vi "AlternativeLauncher.vi"() -> ()   [LabVIEW 2013]
panel:
  out "2nd letter":string
  out "1st letter":string
  out "PASSWORD":string
  out "2nd":bool
  out "1st":bool
  out "Input Signal Energy":dbl
  out "Utterance":dbl[](graph)
  out "Slide":i32(slide) scale=0.0..3000.0
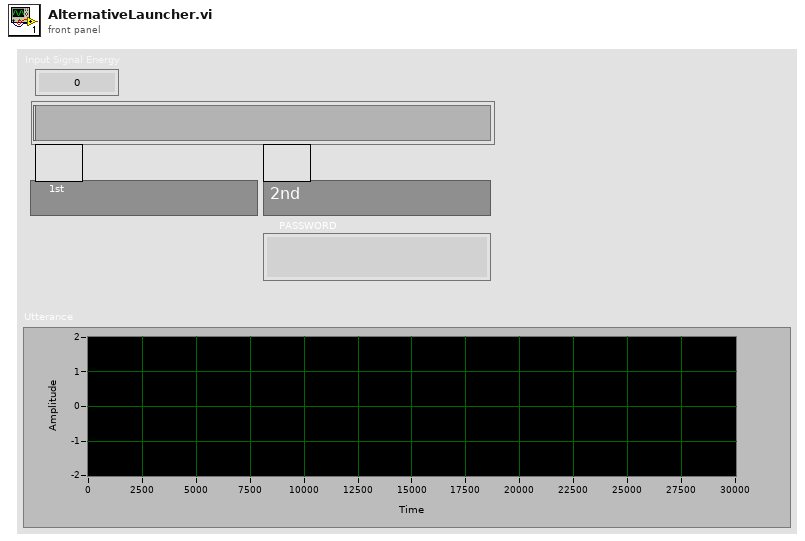
[diagram p1: front panel]
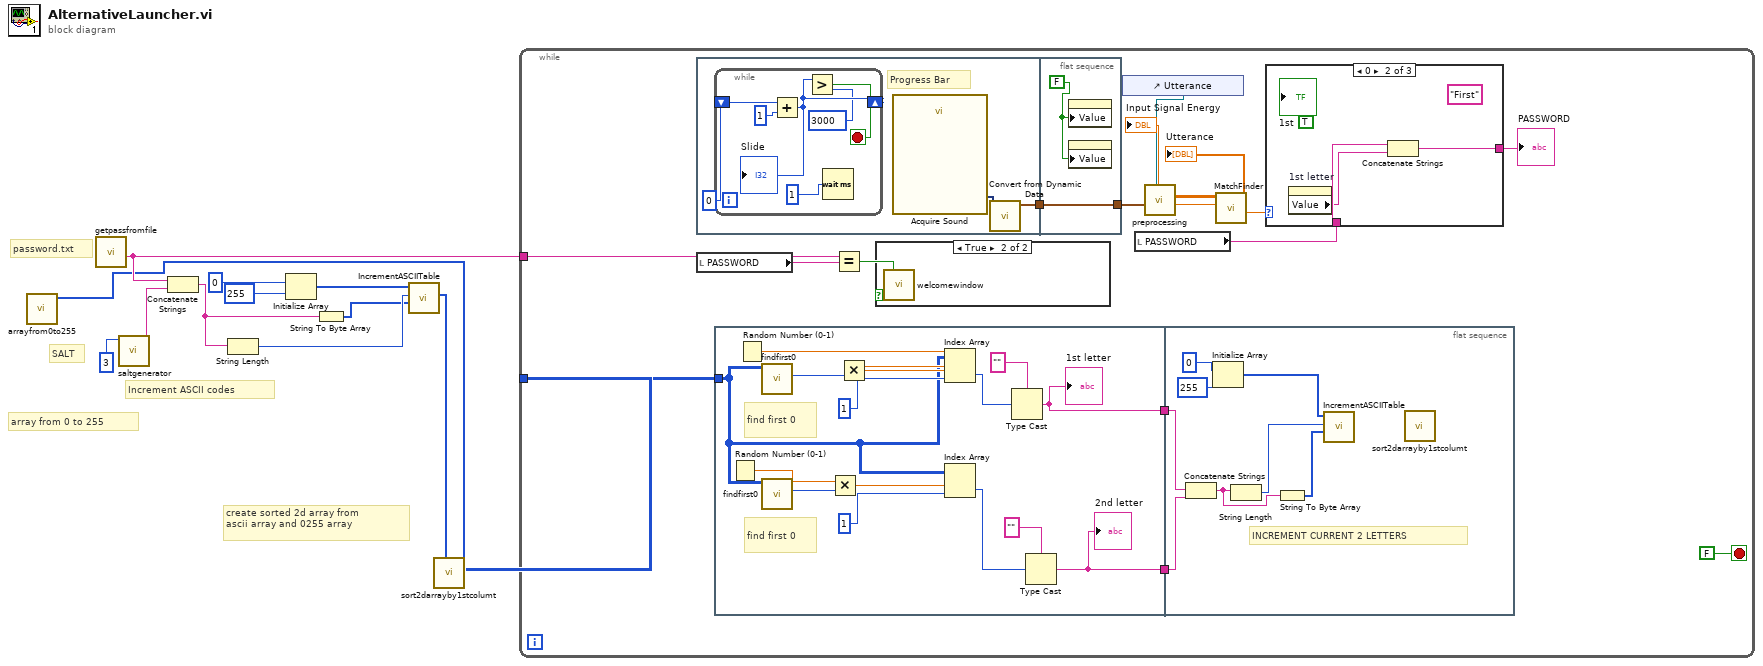
[diagram p0: block diagram]
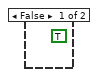
[diagram p2: hidden frame]
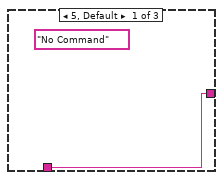
[diagram p3: hidden frame]
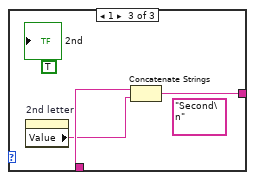
[diagram p4: hidden frame]
diagram:
  # "array from 0 to 255"
  # "create sorted 2d array from \nascii array and 0255 array"
  # "Increment ASCII codes"
  # "SALT"
  # "password.txt"
  n1 = call "arrayfrom0to255.vi"() -> ("Array 2"=w2:i32[])  [unwired: 11 in]
  n2 = call "getpassfromfile.vi"() -> ("line string"=w11:string)  [unwired: 11 in]
  n3 = call "saltgenerator.vi"("Numeric"=3) -> ("string"=w10:string)  [unwired: 10 in]
  n4 = Concatenate Strings(w11, w10) -> (w5:string)
  n5 = String Length(string=w5) -> (length=w6:i32)
  n6 = Initialize Array(0 ("dimension size"), 255 ("dimension size")) -> (w3:i32[])
  n7 = String To Byte Array(string=w5) -> (unsigned byte array=w4:u8[])
  n8 = call "IncrementASCIITable.vi"("0255array"=w4, "Numeric"=w6, "Array in"=w3) -> ("we array"=w9:i32[])  [unwired: 7 in, 1 out]
  n9 = call "sort2darrayby1stcolumt.vi"("array"=w2, "we array"=w9) -> ("Array"=w1:i32[][])  [unwired: 9 in]
  n10 = while {
    tunnel: w11 -> [w18]
    tunnel: w1 -> [w15]
    stop <- FALSE stop-if-true
    n11 = flat-sequence {
      tunnel: [w62] -> w23
      tunnel: [w72] -> w24
      tunnel: w23 -> [w72]
      frame #0 {
        # "Progress Bar"
        n12 = while {
          shift-right: [w67] -> _
          shift-left: 0 -> [w70]
          stop <- w65 stop-if-true
          n13 = Add(x=w70, y=1) -> (x+y=w67:i32)
          "Slide" <- w67
          n14 = Greater?(x=w67, y=u32 3000) -> (0:w65:bool)
          n15 = Wait (ms)(milliseconds to wait=u32 1) -> ()  [unwired: 1 out]
        }
        n16 = call "Acquire Sound"() -> ("Data"=w63:dynamicdata)  [unwired: 18 in, 1 out]
        n17 = call "Convert from Dynamic Data"("Dynamic Data Type"=w63) -> ("Array of Waveform"=w62:waveform(dbl)[])  [unwired: 3 in]
      }
      frame #1 {
        w71 = FALSE ("1st")
        n18 = property class="Bool (strict)"("Value"=w71) -> ()  [unwired: 2 in, 2 out]
        n19 = property class="Bool (strict)"("Value"=w71) -> ()  [unwired: 2 in, 2 out]
      }
    }
    n20 = local read "PASSWORD"() -> (w19:string)
    n21 = flat-sequence {
      tunnel: w15 -> [w36]
      tunnel: [w31] -> w14
      tunnel: [w30] -> w13
      tunnel: w14 -> [w47]
      tunnel: w13 -> [w46]
      frame #0 {
        # "find first 0"
        # "find first 0"
        n22 = Random Number (0-1)() -> (number: 0 to 1=w37:dbl)
        n23 = Random Number (0-1)() -> (number: 0 to 1=w44:dbl)
        n24 = call "findfirst0.vi"("Array"=w36) -> ("index of element"=w43:i32)  [unwired: 10 in]
        n25 = call "findfirst0.vi"("Array"=w36) -> ("index of element"=w38:i32)  [unwired: 10 in]
        n26 = Multiply(x=w37, y=w38) -> (x*y=w40:dbl)
        n27 = Multiply(x=w44, y=w43) -> (x*y=w41:dbl)
        n28 = Index Array(array=w36, index (row)=w41, index (col)=1 ("index (row)")) -> (element=w32:i32)
        n29 = Index Array(array=w36, index (row)=w40, index (col)=1 ("index (row)")) -> (element=w34:i32)
        n30 = Type Cast(type="", x=w32) -> (*(type *) &x=w31:string)
        "1st letter" <- w31
        n31 = Type Cast(type="", x=w34) -> (*(type *) &x=w30:string)
        "2nd letter" <- w30
      }
      frame #1 {
        # "INCREMENT CURRENT 2 LETTERS"
        n32 = Concatenate Strings(w47, w46) -> (w45:string)
        n33 = Initialize Array(0 ("dimension size"), 255 ("dimension size")) -> (w50:i32[])
        n34 = String Length(string=w45) -> (length=w49:i32)
        n35 = String To Byte Array(string=w45) -> (unsigned byte array=w48:u8[])
        n36 = call "IncrementASCIITable.vi"("0255array"=w48, "Numeric"=w49, "Array in"=w50) -> ()  [unwired: 7 in, 2 out]
        n37 = call "sort2darrayby1stcolumt.vi"() -> ()  [unwired: 11 in, 1 out]
      }
    }
    n38 = Equal?(x=w18, y=w19) -> (x = y?=w17:bool)
    n39 = case shown="True" w17 {
      frame False {
        (unwired) TRUE ("Boolean 2")
      }
      frame True {
        n40 = call "welcomewindow.vi"() -> ()  [unwired: 12 in]
      }
    }
    n41 = control-ref of="Utterance"() -> (w26:refnum<vi>)
    n42 = local read "PASSWORD"() -> (w20:string)
    n43 = call "preprocessing.vi"("WaveformGraph in"=w26, "Input Speech"=w24) -> ("Start index"=w29:dbl, "Frames"=w28:dbl[][], "Signal energy"=→"Input Signal Energy":dbl)  [unwired: 6 in, 1 out]
    n44 = call "MatchFinder.vi"("Start index"=w29, "Frames"=w28) -> ("Best Match"=w22:dbl, "Utterance"=→"Utterance":dbl[])  [unwired: 8 in]
    n45 = case shown="0" w22 {
      tunnel: [w53 w56 w60] -> w21
      tunnel: w20 -> [w53 w55 w59]
      frame 5, Default {
        (unwired) "No Command" ("Command")
      }
      frame 0 {
        (unwired) "First" ("Command")
        n46 = property on="1st letter" class="Str"() -> ("Value"=w54:string)  [unwired: 2 in, 2 out]
        n47 = Concatenate Strings(w55, w54) -> (w56:string)
        "1st" <- TRUE ("RIGHT")
      }
      frame 1 {
        (unwired) "Second\n" ("Command")
        n48 = property on="2nd letter" class="Str"() -> ("Value"=w58:string)  [unwired: 2 in, 2 out]
        n49 = Concatenate Strings(w59, w58) -> (w60:string)
        "2nd" <- TRUE ("RIGHT")
      }
    }
    "PASSWORD" <- w21
  }
